vi "SETUPdll_d.vi"(6 "error in (no error)":errorcluster, 7 "Reference State (hrf)":T2, 8 "Path to Mixture file (hfmix)":path=path "C:/Program Files/NIST/RefProp7/fluids/HMX.BNC", 9 "Mixure Cluster in":T1) -> (0 "error out":errorcluster, 3 "Mixure Cluster out":T1)   [LabVIEW 2017]
doc: "Calls the Setupdll function in teh refprop.dll library.\n\nThis funciton must be called before any other calls to the refprop.dll.\n\nAll fluid file and mixture file paths must be absoloute paths.\n\nDeveloped by:\nGreg Sussman\nProcess Automation Corp\nwww.processauto.com\n(267)685-1249"
uses:
  hrf enum_d.ctl
  Mixture Composition cluster_d.ctl
panel:
  out "wm":dbl
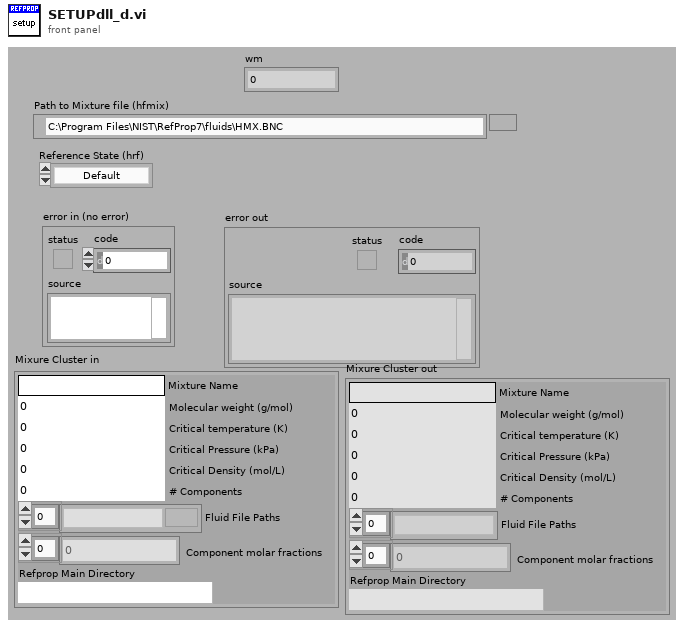
[diagram p1: front panel]
types:
  T1 = typedef "Mixture Composition cluster_d.ctl" = cluster{"Mixture Name":string, "Molecular weight (g/mol)":dbl, "Critical temperature (K)":dbl, "Critical Pressure (kPa)":dbl, "Critical Density (mol/L)":dbl, "# Components":i32, "Fluid File Paths":path[], "Component molar fractions":dbl[], "Refprop Main Directory":path}
  T2 = typedef "hrf enum_d.ctl" = enum16{"Default", "ASHRAE", "IIR"}
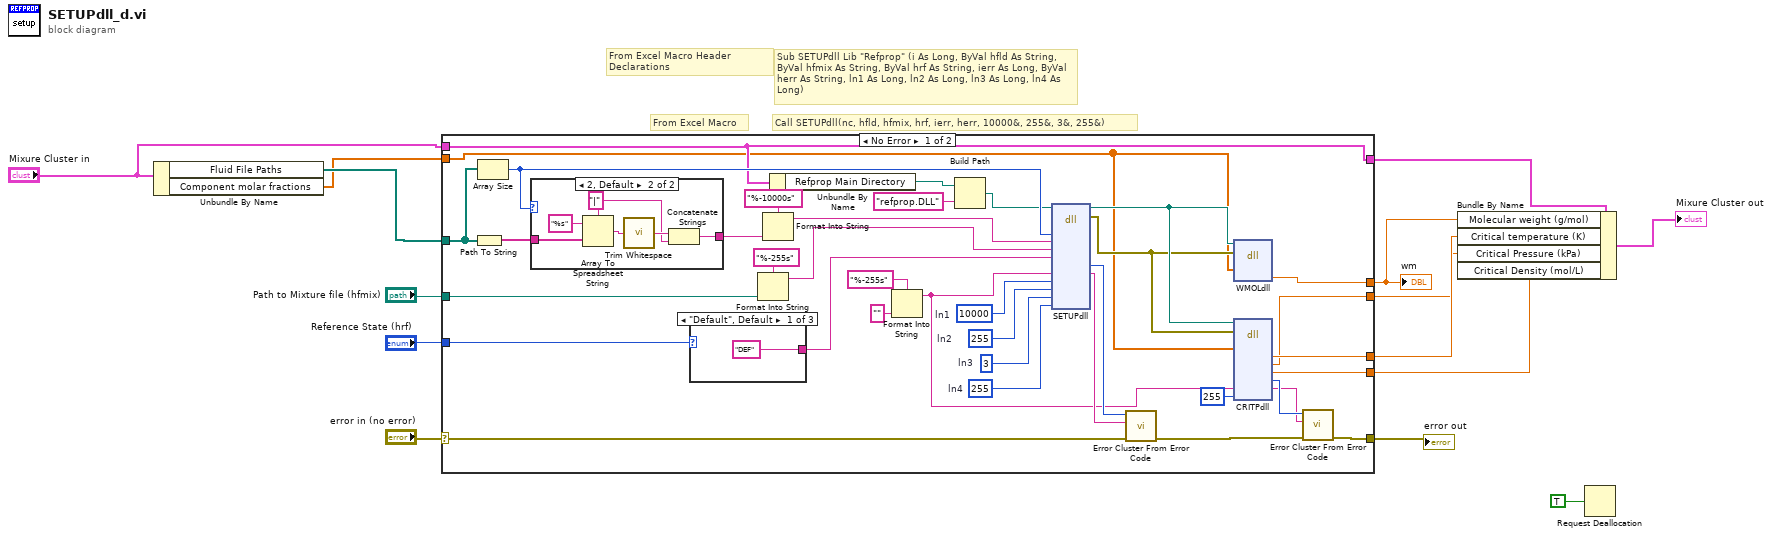
[diagram p0: block diagram]
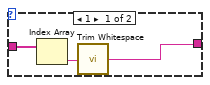
[diagram p2: hidden frame]
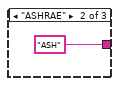
[diagram p3: hidden frame]
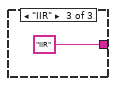
[diagram p4: hidden frame]
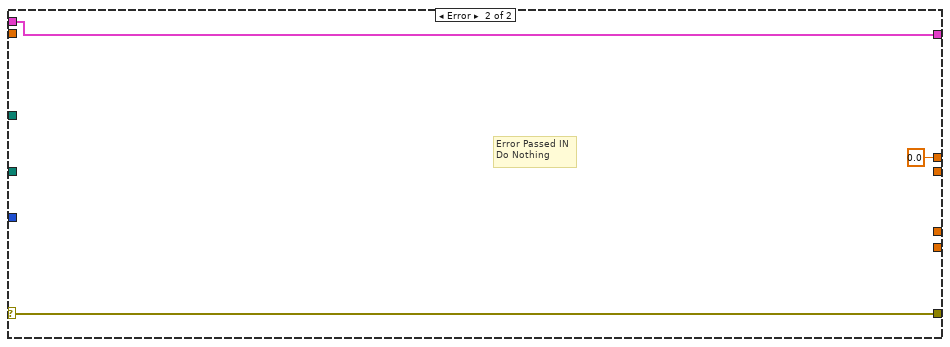
[diagram p5: hidden frame]
diagram:
  # "From Excel Macro"
  # "From Excel Macro Header Declarations"
  # "Sub SETUPdll Lib \"Refprop\" (i As Long, ByVal hfld As String, ByVal hfmix As String, ByVal hrf As String, ierr As Long, ByVal herr As String, ln1 As Long, ln2 As Long, ln3 As Long, ln4 As Long)"
  # "Call SETUPdll(nc, hfld, hfmix, hrf, ierr, herr, 10000&, 255&, 3&, 255&)"
  n1 = Unbundle By Name("Mixure Cluster in") -> ("Fluid File Paths"=w10:path[], "Component molar fractions"=w9:dbl[])
  n2 = case shown="No Error" "error in (no error)" {
    selector: "error in (no error)" -> [w38 w66]
    tunnel: "Path to Mixture file (hfmix)" -> [w45 _]
    tunnel: [w19 w66] -> w13
    tunnel: "Reference State (hrf)" -> [w40 _]
    tunnel: w10 -> [w34 _]
    tunnel: w9 -> [w24 _]
    tunnel: [w31 0.0 ("wm")] -> w7
    tunnel: "Mixure Cluster in" -> [w30 w64]
    tunnel: [w30 w64] -> w6
    tunnel: [w23 _] -> w3
    tunnel: [w22 _] -> w2
    tunnel: [w21 _] -> w1
    frame No Error {
      w48 = 255  # ln4
      w49 = 3  # ln3
      w50 = 255  # ln2
      w51 = 10000  # ln1
      n3 = Path To String(path=w34) -> (string=w35:string[])
      n4 = Array Size(array=w34) -> (size(s)=w33:i32)
      n5 = case shown="2, Default" w33 {
        tunnel: [w52 w57] -> w36
        tunnel: w35 -> [w54 w56]
        frame 1 {
          n6 = Index Array(array=w54) -> (element=w53:string)  [unwired: 1 in]
          n7 = call <vilib>:"Trim Whitespace.vi"("string"=w53) -> ("trimmed string"=w52:string)  [unwired: 1 in]
        }
        frame 2, Default {
          w55 = "|"
          n8 = Array To Spreadsheet String(delimiter (Tab)=w55, array=w56, 3:"%s" ("format string")) -> (spreadsheet string=w59:string)
          n9 = call <vilib>:"Trim Whitespace.vi"("string"=w59) -> ("trimmed string"=w60:string)  [unwired: 1 in]
          n10 = Concatenate Strings(w60, w55) -> (w57:string)
        }
      }
      n11 = case shown="\"Default\", Default" w40 {
        tunnel: ["DEF" "ASH" "IIR"] -> w39
        frame "Default", Default {
        }
        frame "ASHRAE" {
        }
        frame "IIR" {
        }
      }
      n12 = Format Into String(format string="%-255s", w45) -> (resulting string=w44:string)  [unwired: 2 in, 1 out]
      n13 = Format Into String(format string="%-10000s", w36) -> (resulting string=w37:string)  [unwired: 2 in, 1 out]
      n14 = Unbundle By Name(w30) -> ("Refprop Main Directory"=w29:path)
      n15 = Format Into String(format string="%-255s", "") -> (resulting string=w16:string)  [unwired: 2 in, 1 out]
      n16 = Build Path(base path=w29, name or relative path="refprop.DLL" ("名称或相对路径")) -> (appended path=w28:path)
      n17 = dll-call lib="C:/Program Files (x86)/National Instruments/LabVIEW 2017/user.lib/REFPROP/refprop.dll" fn="SETUPdll"(path in=w28, "i"=w33, "hfld"=w37, "hfmix"=w44, "hrf"=w39, "herr"=w16, "ln1"=w51, "ln2"=w50, "ln3"=w49, "ln4"=w48) -> (path out=w26:path, error out=w25:errorcluster, "ierr"=w32:i32, "herr"=w41:string)  [unwired: 12 in]
      n18 = call <vilib>:"Error Cluster From Error Code.vi"("error in (no error)"=w38, "error message (\"\")"=w41, "error code (0)"=w32) -> ("error out"=w20:errorcluster)  [unwired: 6 in]
      n19 = dll-call lib="refprop.DLL" fn="WMOLdll"(path in=w26, error in=w25, "x1"=w24) -> ("wm"=w31:dbl)  [unwired: 4 in, 2 out]
      n20 = dll-call lib="C:/Program Files (x86)/National Instruments/LabVIEW 2017/user.lib/REFPROP/refprop.dll" fn="CRITPdll"(path in=w26, error in=w25, "z"=w24, "herr"=w16, "herr_length"=255) -> ("Tc"=w23:dbl, "Pc"=w22:dbl, "Dc"=w21:dbl, "ierr"=w18:i32, "herr"=w17:string)  [unwired: 8 in, 2 out]
      n21 = call <vilib>:"Error Cluster From Error Code.vi"("error in (no error)"=w20, "error message (\"\")"=w17, "error code (0)"=w18) -> ("error out"=w19:errorcluster)  [unwired: 6 in]
    }
    frame Error {
      # "Error Passed IN\nDo Nothing"
    }
  }
  "error out" <- w13
  "wm" <- w7
  n22 = Bundle By Name(cluster=w6, "Molecular weight (g/mol)"=w7, "Critical temperature (K)"=w3, "Critical Pressure (kPa)"=w2, "Critical Density (mol/L)"=w1) -> (→"Mixure Cluster out":T1)
  n23 = Request Deallocation(TRUE ("标志")) -> ()
